vi "LabVIEW.vi"() -> ()   [LabVIEW 2014]
panel:
  in  "VIs":T1(array[cluster])
  out "LabVIEW":refnum<vi>
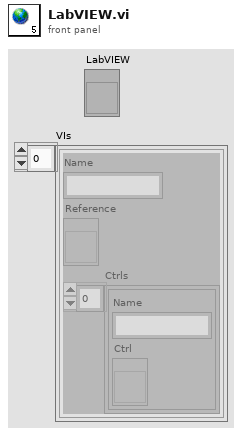
[diagram p1: front panel]
types:
  T1 = cluster{"Name":string, "Reference":refnum<vi>, "Ctrls":cluster{"Name":string, "Ctrl":refnum<vi>}[]}[]
diagram:
